vi "Email Handler (PC).vi"() -> ()   [LabVIEW 2019]
uses:
  Type Defs/Email Cluster v2.ctl
  Controls/Alarm Config.ctl
  Controls/Alarm Definition.ctl
  Controls/Alarm Profile Config.ctl
panel:
  in  "Boolean":bool
  out "Tab Control":enum32{"Page 1", "Page 2"}(tab)
  in  "Emails":T1[](array[typedef])
  out "Unsent Emails":i32
  in  "Script Path":path=path "C:/Projects/Alarm Email Handler/Executable/Script/gmail_script.py"
  in  "Path to Python.exe":path=path "C:/Python35-32/python.exe"
  # "Keep Running & Minimized"
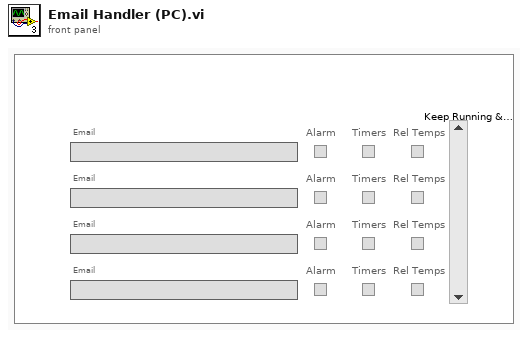
[diagram p1: front panel]
types:
  T1 = typedef "Email Cluster v2.ctl" = cluster{"Email":string, "Alarm":bool, "Timers":bool, "Rel Temps":bool}
  T2 = cluster{"ArmedAddresses":i32[], "Tracker":i32, "Armed":bool, "Emails":T1[], "Alarm":bool, "Unsent Emails":i32, "IP to Check":i32, "Email Data":string[], "Email Config Path":path}
  T3 = enum16{"open", "replace", "create", "open or create", "replace or create", "replace or create with confirmation"}
  T4 = typedef "Alarm Config.ctl" = cluster{"Alarms:":T5[], "Profile Sync:":T6}
  T5 = typedef "Alarm Definition.ctl" = cluster{"Description:":string, "Enabled:":bool, "Data Index:":i32, "Data Type:":string, "Low Limit:":dbl, "High Limit:":dbl, "Trip Time:":u32, "Profile Sync:":bool}
  T6 = typedef "Alarm Profile Config.ctl" = cluster{"Trip Time:":u32, "Consecutive Trips:":i32}
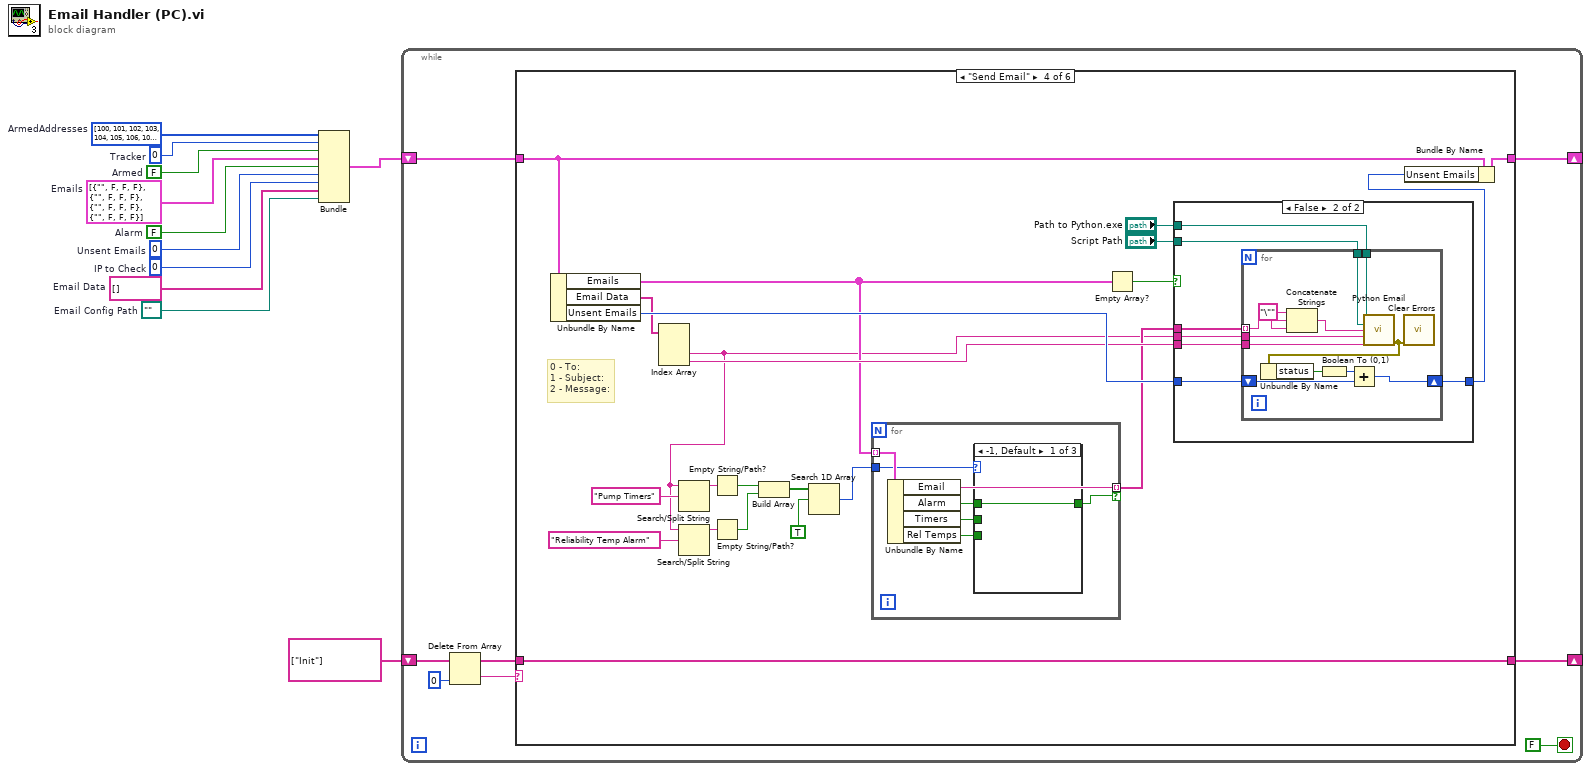
[diagram p0: block diagram]
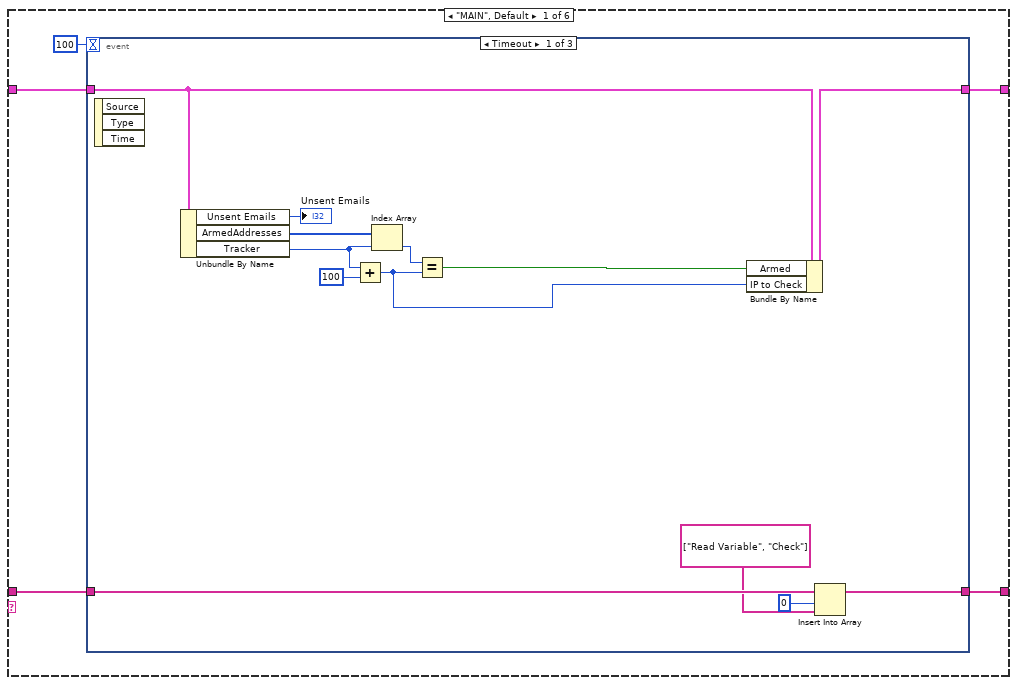
[diagram p2: hidden frame]
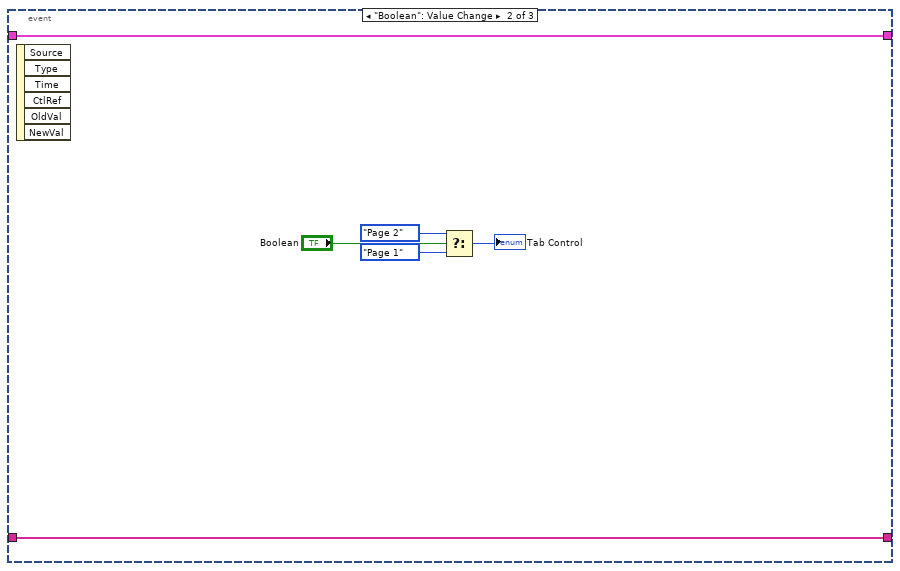
[diagram p3: hidden frame]
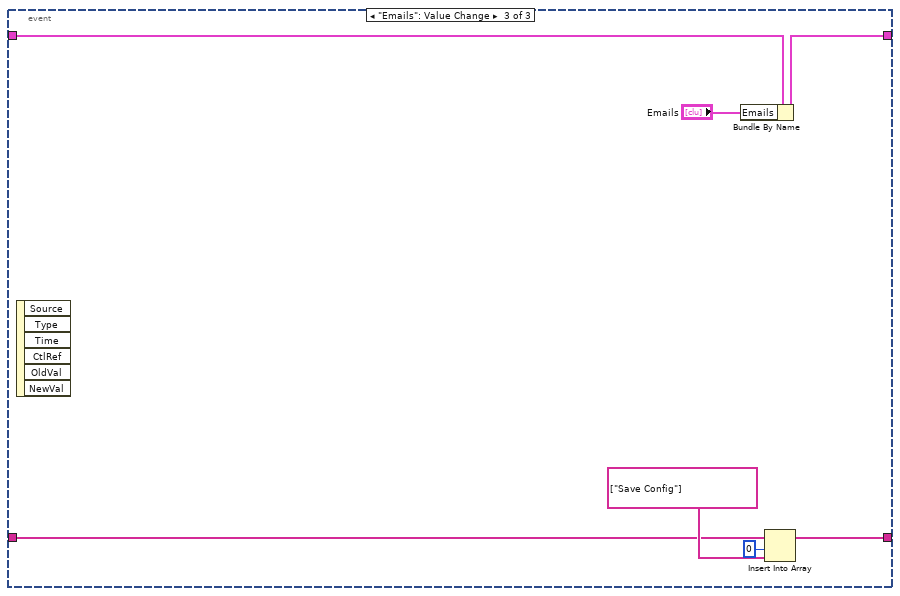
[diagram p4: hidden frame]
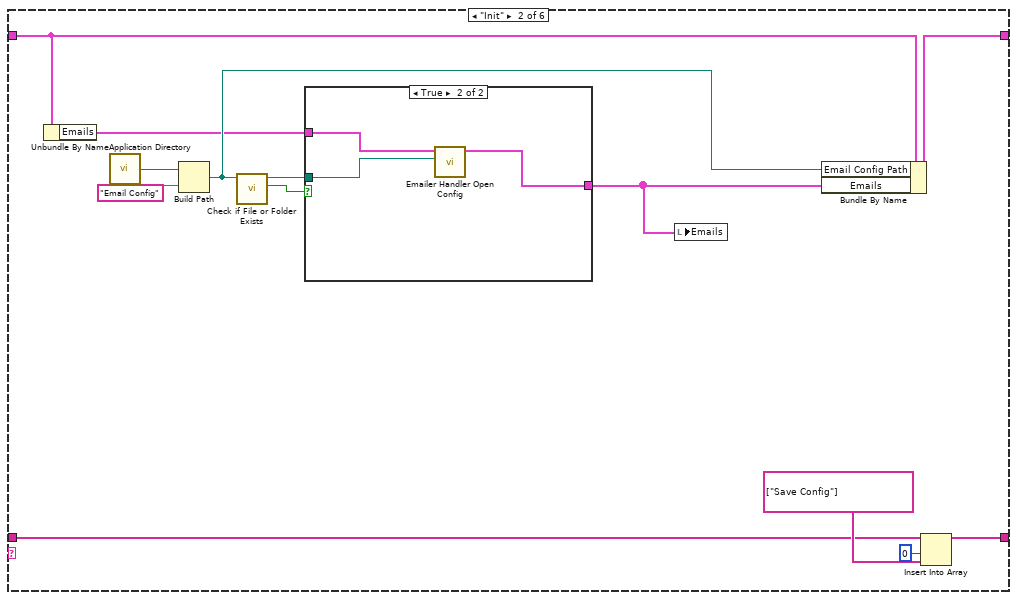
[diagram p5: hidden frame]
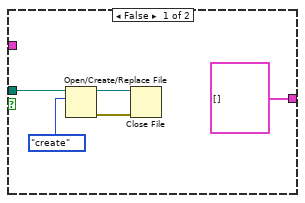
[diagram p6: hidden frame]
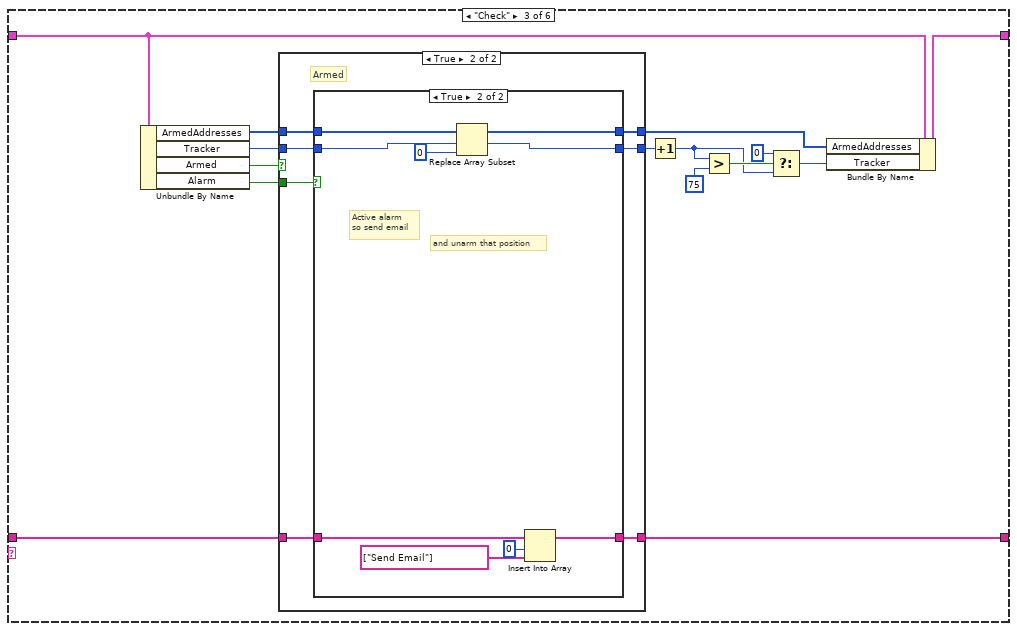
[diagram p7: hidden frame]
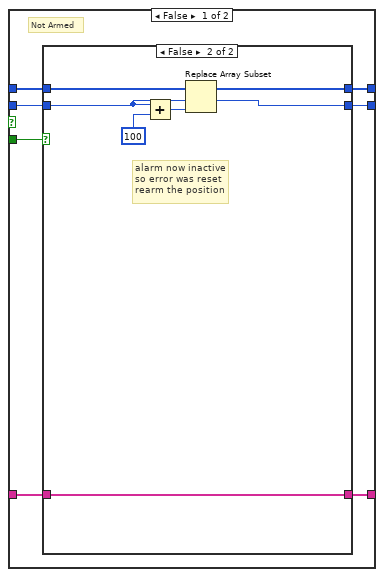
[diagram p8: hidden frame]
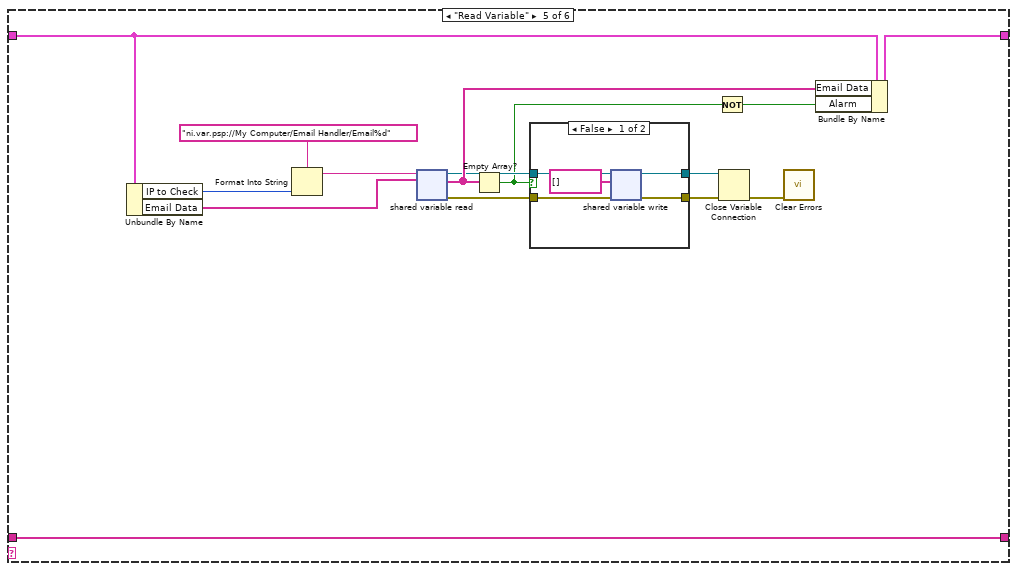
[diagram p14: hidden frame]
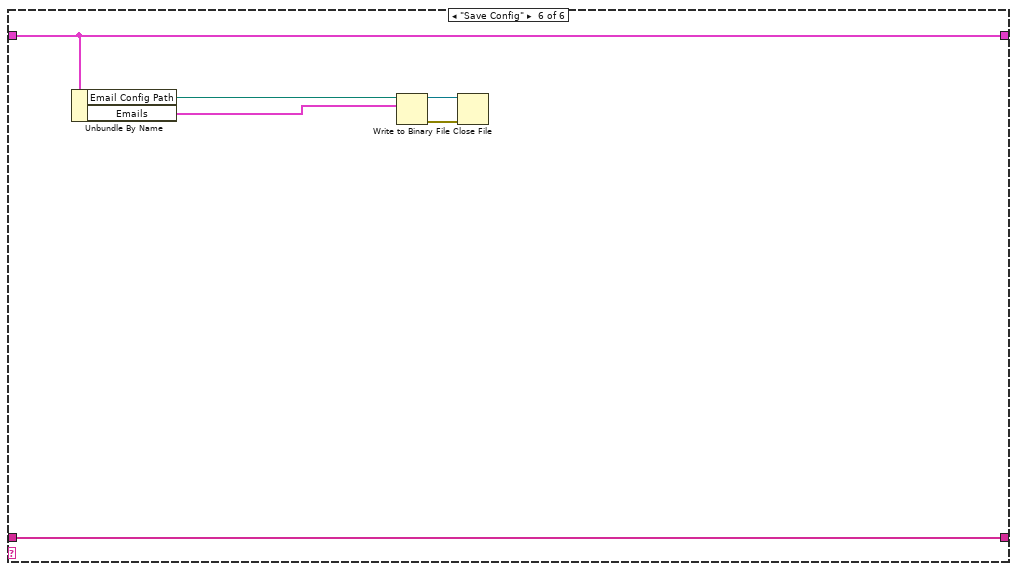
[diagram p16: hidden frame]
diagram:
  w1 = T1[] [{"Email"="", "Alarm"=FALSE, "Timers"=FALSE, "Rel Temps"=FALSE}, {"Email"="", "Alarm"=FALSE, "Timers"=FALSE, "Rel Temps"=FALSE}, {"Email"="", "Alarm"=FALSE, "Timers"=FALSE, "Rel Temps"=FALSE}, {"Email"="", "Alarm"=FALSE, "Timers"=FALSE, "Rel Temps"=FALSE}]  # Emails
  w2 = path ""  # Email Config Path
  w3 = string[] []  # Email Data
  w4 = 0  # IP to Check
  w5 = 0  # Unsent Emails
  w6 = FALSE  # Alarm
  w7 = FALSE  # Armed
  w9 = i32[] [100, 101, 102, 103, 104, 105, 106, 107, 108, 109, 110, 111, 112, 113, 114, 115, 116, 117, 118, 119, 120, 121, 122, 123, 124, 125, 126, 127, 128, 129, 130, 131, 132, 133, 134, 135, 136, 137, 138, 139, 140, 141, 142, 143, 144, 145, 146, 147, 148, 149, 150, 151, 152, 153, 154, 155, 156, 157, 158, 159, 160, 161, 162, 163, 164, 165, 166, 167, 168, 169, 170, 171, 172, 173, 174, 175]  # ArmedAddresses
  w11 = 0  # Tracker
  n1 = Bundle("ArmedAddresses"=w9, "Tracker"=w11, "Armed"=w7, "Emails"=w1, "Alarm"=w6, "Unsent Emails"=w5, "IP to Check"=w4, "Email Data"=w3, "Email Config Path"=w2) -> (w10:T2)  [unwired: 1 in]
  n2 = while {
    shift-right: [w12] -> _
    shift-left: w10 -> [w18]
    shift-right: [w13] -> _
    shift-left: string[] ["Init"] -> [w17]
    stop <- FALSE stop-if-true
    n3 = Delete From Array(array=w17, index=0) -> (deleted portion=w15:string, array with subset deleted=w14:string[])  [unwired: 1 in]
    n4 = case shown="\"Send Email\"" w15 {
      tunnel: w18 -> [w24 w56 w81 w140 w185 w198]
      tunnel: w14 -> [w22 w52 w78 w142 w187 w200]
      tunnel: [w21 w51 w75 w142 w187 w200] -> w13
      tunnel: [w23 w59 w80 w139 w186 w198] -> w12
      frame "MAIN", Default {
        n5 = event shown="[0] Timeout" {
          selector: _ -> [_ _ _]
          dyn-events: _ -> [_ _ _]
          timeout: 100 -> [_ _ _]
          tunnel: w24 -> [w36 w39 w50]
          tunnel: [w35 w39 w49] -> w23
          tunnel: w22 -> [w31 w38 w44]
          tunnel: [w27 w38 w45] -> w21
          event Timeout {
            n6 = event-data() -> ()  [unwired: 1 in, 3 out]
            n7 = Unbundle By Name(w36) -> ("Unsent Emails"=→"Unsent Emails":i32, "ArmedAddresses"=w37:i32[], "Tracker"=w30:i32)
            n8 = Add(x=w30, y=100) -> (x+y=w28:i32)
            n9 = Index Array(array=w37, index=w30) -> (element=w33:i32)
            n10 = Equal?(x=w33, y=w28) -> (x = y?=w32:bool)
            n11 = Bundle By Name(cluster=w36, "Armed"=w32, "IP to Check"=w28) -> (w35:T2)
            n12 = Insert Into Array(array=w31, index=0, new element=string[] ["Read Variable", "Check"]) -> (w27:string[])
          }
          event "Boolean": Value Change {
            n13 = event-data() -> ()  [unwired: 1 in, 6 out]
            n14 = Select(t=enum32{"Page 1", "Page 2"}."Page 2" ("Tab Control"), s="Boolean", f=enum32{"Page 1", "Page 2"}."Page 1" ("Tab Control")) -> (s? t:f=→"Tab Control":enum32{"Page 1", "Page 2"})
          }
          event "Emails": Value Change {
            n15 = event-data() -> ()  [unwired: 1 in, 6 out]
            n16 = Bundle By Name(cluster=w50, "Emails"="Emails") -> (w49:T2)
            n17 = Insert Into Array(array=w44, index=0, new element=string[] ["Save Config"]) -> (w45:string[])
          }
        }
      }
      frame "Init" {
        n18 = Unbundle By Name(w56) -> ("Emails"=w55:T1[])
        n19 = call <vilib>:"Application Directory.vi"() -> ("Application Directory"=w61:path)
        n20 = Build Path(base path=w61, name or relative path="Email Config") -> (appended path=w58:path)
        n21 = call <vilib>:"Check if File or Folder Exists.vi"("path"=w58) -> ("file or folder exists?"=w62:bool, "dup path"=w63:path)  [unwired: 8 in, 1 out]
        n22 = case shown="True" w62 {
          tunnel: w63 -> [w67 w69]
          tunnel: [T1[] [] ("Emails") w71] -> w57
          tunnel: w55 -> [_ w70]
          frame False {
            (unwired) T4 {"Alarms:"=[{"Description:"="", "Enabled:"=FALSE, "Data Index:"=0, "Data Type:"="", "Low Limit:"=0.0, "High Limit:"=0.0, "Trip Time:"=0, "Profile Sync:"=FALSE}, {"Description:"="", "Enabled:"=FALSE, "Data Index:"=0, "Data Type:"="", "Low Limit:"=0.0, "High Limit:"=0.0, "Trip Time:"=0, "Profile Sync:"=FALSE}, {"Description:"="", "Enabled:"=FALSE, "Data Index:"=0, "Data Type:"="", "Low Limit:"=0.0, "High Limit:"=0.0, "Trip Time:"=0, "Profile Sync:"=FALSE}, {"Description:"="", "Enabled:"=FALSE, "Data Index:"=0, "Data Type:"="", "Low Limit:"=0.0, "High Limit:"=0.0, "Trip Time:"=0, "Profile Sync:"=FALSE}, {"Description:"="", "Enabled:"=FALSE, "Data Index:"=0, "Data Type:"="", "Low Limit:"=0.0, "High Limit:"=0.0, "Trip Time:"=0, "Profile Sync:"=FALSE}, {"Description:"="", "Enabled:"=FALSE, "Data Index:"=0, "Data Type:"="", "Low Limit:"=0.0, "High Limit:"=0.0, "Trip Time:"=0, "Profile Sync:"=FALSE}, {"Description:"="", "Enabled:"=FALSE, "Data Index:"=0, "Data Type:"="", "Low Limit:"=0.0, "High Limit:"=0.0, "Trip Time:"=0, "Profile Sync:"=FALSE}, {"Description:"="", "Enabled:"=FALSE, "Data Index:"=0, "Data Type:"="", "Low Limit:"=0.0, "High Limit:"=0.0, "Trip Time:"=0, "Profile Sync:"=FALSE}], "Profile Sync:"={"Trip Time:"=0, "Consecutive Trips:"=0}} ("Alarm Config")
            n23 = Open/Create/Replace File(file path (use dialog)=w67, operation (0:open)=T3."create") -> (refnum out=w66:refnum<file>, error out=w65:errorcluster)  [unwired: 4 in, 1 out]
            n24 = Close File(refnum=w66, error in=w65) -> ()  [unwired: 2 out]
          }
          frame True {
            n25 = call "Emailer Handler Open Config.vi"("Config Path"=w69, "Emails IN"=w70) -> ("Emails OUT"=w71:T1[])  [unwired: 9 in]
          }
        }
        n26 = local write "Emails"(w57) -> ()
        n27 = Bundle By Name(cluster=w56, "Email Config Path"=w58, "Emails"=w57) -> (w59:T2)
        n28 = Insert Into Array(array=w52, index=0, new element=string[] ["Save Config"]) -> (w51:string[])
      }
      frame "Check" {
        n29 = Unbundle By Name(w81) -> ("ArmedAddresses"=w74:i32[], "Tracker"=w77:i32, "Armed"=w79:bool, "Alarm"=w72:bool)
        n30 = case shown="True" w79 {
          tunnel: w78 -> [w93 w109]
          tunnel: w77 -> [w90 w106]
          tunnel: [w87 w103] -> w76
          tunnel: w72 -> [w89 w107]
          tunnel: [w92 w108] -> w75
          tunnel: w74 -> [w91 w105]
          tunnel: [w88 w104] -> w73
          frame False {
            # "Not Armed"
            n31 = case shown="False" w89 {
              tunnel: w93 -> [w94 w97]
              tunnel: [w94 w97] -> w92
              tunnel: w90 -> [w95 w100]
              tunnel: w91 -> [w96 w102]
              tunnel: [w96 w101] -> w88
              tunnel: [w95 w100] -> w87
              frame True {
                # "Alarm still active\nerror has not been reset\nleave unarmed"
              }
              frame False {
                # "alarm now inactive\nso error was reset\nrearm the position"
                n32 = Add(x=w100, y=100) -> (x+y=w99:i32)
                n33 = Replace Array Subset(array=w102, new element=w99, index=w100) -> (w101:i32[])
              }
            }
          }
          frame True {
            # "Armed"
            n34 = case shown="True" w107 {
              tunnel: w109 -> [w110 w120]
              tunnel: [w110 w119] -> w108
              tunnel: w106 -> [w111 w114]
              tunnel: w105 -> [w112 w116]
              tunnel: [w112 w115] -> w104
              tunnel: [w111 w114] -> w103
              frame False {
                # "No Alarm"
              }
              frame True {
                # "and unarm that position"
                # "Active alarm\nso send email"
                n35 = Replace Array Subset(array=w116, new element=0, index=w114) -> (w115:i32[])
                n36 = Insert Into Array(array=w120, index=0, new element=string[] ["Send Email"]) -> (w119:string[])
              }
            }
          }
        }
        n37 = Increment(x=w76) -> (x+1=w83:i32)
        n38 = Greater?(x=w83, y=75) -> (0:w85:bool)
        n39 = Select(t=0, s=w85, f=w83) -> (s? t:f=w82:i32)
        n40 = Bundle By Name(cluster=w81, "ArmedAddresses"=w73, "Tracker"=w82) -> (w80:T2)
      }
      frame "Send Email" {
        # "0 - To:\n1 - Subject:\n2 - Message:"
        n41 = Unbundle By Name(w140) -> ("Emails"=w132:T1[], "Email Data"=w137:string[], "Unsent Emails"=w141:i32)
        n42 = Index Array(array=w137) -> (element #2=w121:string, element #3=w136:string)  [unwired: 3 in, 1 out]
        n43 = Search/Split String(string=w121, search string/char (-)="Pump Timers") -> (substring before match=w130:string)  [unwired: 1 in, 2 out]
        n44 = Search/Split String(string=w121, search string/char (-)="Reliability Temp Alarm") -> (substring before match=w129:string)  [unwired: 1 in, 2 out]
        n45 = Empty String/Path?(string/path=w130) -> (empty?=w127:bool)
        n46 = Empty String/Path?(string/path=w129) -> (empty?=w126:bool)
        n47 = Build Array(w127, w126) -> (w125:bool[])
        n48 = Search 1D Array(1D array=w125, element=TRUE) -> (index of element=w123:i32)  [unwired: 1 in]
        n49 = for {
          tunnel: w132 -> [w149] mode=indexing
          tunnel: w123 -> [w148]
          tunnel: [w147] -> w122 mode=indexing if=w145
          n50 = Unbundle By Name(w149) -> ("Email"=w147:string, "Alarm"=w146:bool, "Timers"=w144:bool, "Rel Temps"=w143:bool)
          n51 = case shown="-1, Default" w148 {
            tunnel: [w150 w151 w152] -> w145
            tunnel: w146 -> [w150 _ _]
            tunnel: w144 -> [_ w151 _]
            tunnel: w143 -> [_ _ w152]
            frame -1, Default {
            }
            frame 0 {
            }
            frame 1 {
            }
          }
        }
        n52 = Empty Array?(array=w132) -> (empty?=w135:bool)
        n53 = case shown="False" w135 {
          tunnel: w136 -> [_ w155]
          tunnel: w121 -> [_ w156]
          tunnel: w122 -> [_ w160]
          tunnel: w141 -> [w153 w159]
          tunnel: [w153 w154] -> w138
          tunnel: "Path to Python.exe" -> [_ w158]
          tunnel: "Script Path" -> [_ w157]
          frame True {
          }
          frame False {
            n54 = for {
              tunnel: w160 -> [w169] mode=indexing
              tunnel: w156 -> [w172]
              tunnel: w155 -> [w171]
              shift-right: [w164] -> w154
              shift-left: w159 -> [w166]
              tunnel: w158 -> [w162]
              tunnel: w157 -> [w161]
              w170 = "\"" ("string")
              n55 = Concatenate Strings(w170, w169, w170) -> (w168:string)
              n56 = call "Python Email.vi"("Path to Python.exe"=w162, "Script Path"=w161, "To:"=w168, "Subject:"=w172, "Message:"=w171) -> ("error out"=w163:errorcluster)  [unwired: 6 in, 4 out]
              n57 = Unbundle By Name(w163) -> ("status"=w167:bool)
              n58 = Boolean To (0,1)(Boolean=w167) -> (0, 1=w165:i16)
              n59 = Add(x=w165, y=w166) -> (x+y=w164:i32)
              n60 = call <vilib>:"Clear Errors.vi"("error in (no error)"=w163) -> ()  [unwired: 5 in, 2 out]
            }
          }
        }
        n61 = Bundle By Name(cluster=w140, "Unsent Emails"=w138) -> (w139:T2)
      }
      frame "Read Variable" {
        n62 = Unbundle By Name(w185) -> ("IP to Check"=w183:i32, "Email Data"=w181:string[])
        n63 = Format Into String(format string="ni.var.psp://My Computer/Email Handler/Email%d", w183) -> (resulting string=w182:string)  [unwired: 2 in, 1 out]
        n64 = shared-variable-read(w182, w181) -> (w179:refnum<k21>, w178:errorcluster, w180:string[])  [unwired: 1 in, 1 out]
        n65 = Empty Array?(array=w180) -> (empty?=w175:bool)
        n66 = case shown="False" w175 {
          tunnel: w179 -> [w192 w194]
          tunnel: w178 -> [w191 w193]
          tunnel: [w189 w194] -> w177
          tunnel: [w188 w193] -> w176
          frame False {
            n67 = shared-variable-write(w192, w191, string[] [] ("data in")) -> (w189:refnum<k21>, w188:errorcluster)
          }
          frame True {
          }
        }
        n68 = Not(x=w175) -> (.not. x?=w173:bool)
        n69 = Close Variable Connection(8:w176, 11:w177) -> (0:w174:errorcluster)
        n70 = call <vilib>:"Clear Errors.vi"("error in (no error)"=w174) -> ()  [unwired: 5 in, 2 out]
        n71 = Bundle By Name(cluster=w185, "Email Data"=w180, "Alarm"=w173) -> (w186:T2)
      }
      frame "Save Config" {
        n72 = Unbundle By Name(w198) -> ("Email Config Path"=w199:path, "Emails"=w197:T1[])
        n73 = Write to Binary File(file (use dialog)=w199, data=w197) -> (refnum out=w196:refnum<file>, error out=w195:errorcluster)  [unwired: 4 in, 1 out]
        n74 = Close File(refnum=w196, error in=w195) -> ()  [unwired: 2 out]
      }
    }
  }
